vi "Arm movements Sub VI.vi"(11 "BrickReference in":T1) -> (3 "BrickReference out":T1)   [LabVIEW 2016]
uses:
  <vilib>/NXT/Subs/LVHSConnector.ctl
  <vilib>/NXT/LegoClasses/BrickReference/BrickReference.lvclass
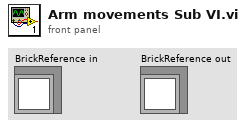
[diagram p1: front panel]
types:
  T1 = typedef "LVHSConnector.ctl" = refnum<class "BrickReference.lvclass">
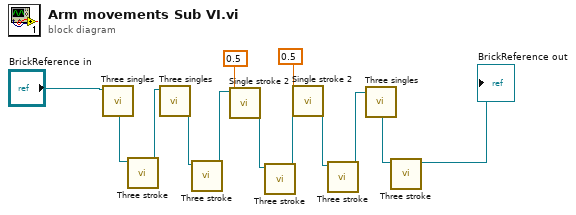
[diagram p0: block diagram]
diagram:
  n1 = call "Three singles.vi"("BrickReference in"="BrickReference in") -> ("BrickReference out"=w1:T1)  [unwired: 10 in]
  n2 = call "Three stroke.vi"("BrickReference in"=w1) -> ("BrickReference out"=w2:T1)  [unwired: 10 in]
  n3 = call "Three singles.vi"("BrickReference in"=w2) -> ("BrickReference out"=w3:T1)  [unwired: 10 in]
  n4 = call "Three stroke.vi"("BrickReference in"=w3) -> ("BrickReference out"=w4:T1)  [unwired: 10 in]
  n5 = call "Single stroke 2.vi"("Numeric"=0.5, "BrickReference in"=w4) -> ("BrickReference out"=w5:T1)  [unwired: 9 in]
  n6 = call "Three stroke.vi"("BrickReference in"=w5) -> ("BrickReference out"=w7:T1)  [unwired: 10 in]
  n7 = call "Single stroke 2.vi"("Numeric"=0.5, "BrickReference in"=w7) -> ("BrickReference out"=w6:T1)  [unwired: 9 in]
  n8 = call "Three stroke.vi"("BrickReference in"=w6) -> ("BrickReference out"=w9:T1)  [unwired: 10 in]
  n9 = call "Three singles.vi"("BrickReference in"=w9) -> ("BrickReference out"=w8:T1)  [unwired: 10 in]
  n10 = call "Three stroke.vi"("BrickReference in"=w8) -> ("BrickReference out"=→"BrickReference out":T1)  [unwired: 10 in]
